vi "Set AppName.vi"(8 "error in (no error)":errorcluster, 10 "AppName":string, 11 "ErrorHandler in":refnum<class "ErrorHandler.lvclass">) -> (0 "error out":errorcluster, 3 "ErrorHandler out":refnum<class "ErrorHandler.lvclass">)   [LabVIEW 2017, in "ErrorHandler.lvclass"]
doc: "Developed by Kevin Thompson\nkevin@thompsonengineering.net\n\nCopyright 2018\nThompson Engineering, LLC"
uses:
  ErrorHandler.lvclass
  ErrorHandler.lvclass/ErrorHandler.ctl
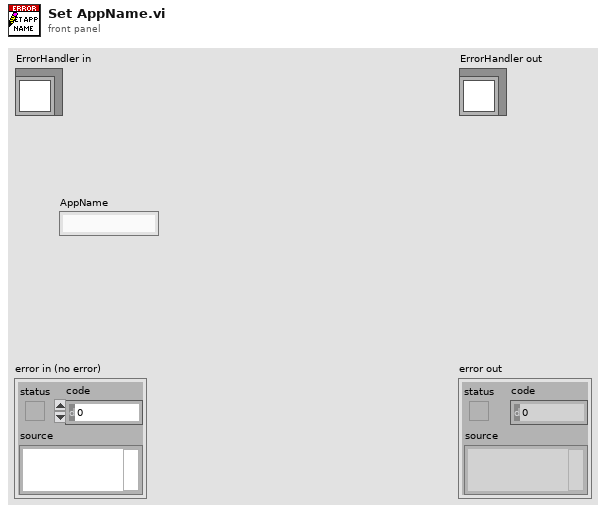
[diagram p1: front panel]
types:
  T1 = typedef "ErrorHandler.lvclass/ObjData--cluster.ctl" = cluster{"AppName":string, "ErrorLogBasePath":path, "ErrorDialogPopUp Disabled":bool, "TerminateAppOnError Enabled":bool}
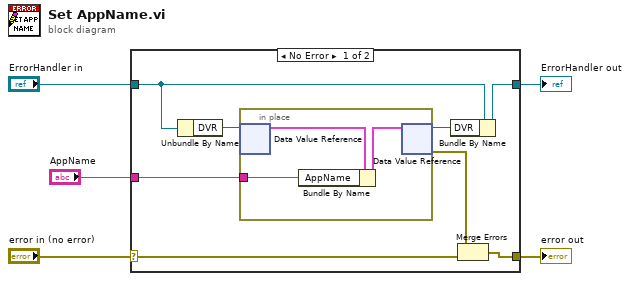
[diagram p0: block diagram]
diagram:
  n1 = case shown="No Error" "error in (no error)" {
    selector: "error in (no error)" -> [w13 w17]
    tunnel: [w8 w17] -> w4
    tunnel: [w10 w18] -> w2
    tunnel: "ErrorHandler in" -> [w9 w18]
    tunnel: "AppName" -> [w12 _]
    frame No Error {
      n2 = Unbundle By Name(w9) -> ("DVR"=w6:refnum<data-value>)
      n3 = in-place {
        in-place-border: w12 -> [w16]
        n4 = in-place-dvr #1(w6) -> (w15:T1)  [unwired: 1 out]
        n5 = Bundle By Name(cluster=w15, "AppName"=w16) -> (w14:T1)
        n6 = in-place-dvr #1(w14) -> (w11:refnum<data-value>, w7:errorcluster)
      }
      n7 = Bundle By Name(cluster=w9, "DVR"=w11) -> (w10:refnum<class "ErrorHandler.lvclass">)
      n8 = Merge Errors(w7, w13) -> (w8:errorcluster)
    }
    frame Error {
    }
  }
  "error out" <- w4
  "ErrorHandler out" <- w2
